vi "CraciunAlexandru_ChelaruIoana_FSM_3a (1).vi"() -> ()   [LabVIEW 2021]
uses:
  <vilib>/Skyline/Tag/Shared/typedefs/DataType.ctl
  <vilib>/Skyline/Configuration/Configuration HTTP_class/Open Configuration HTTP Auto.vi
  <vilib>/Skyline/Tag/Wrapper/Wrapper_class/Write Tag (I32).vi
  <vilib>/Skyline/Tag/Wrapper/Wrapper HTTP_class/NI Skyline Tag HTTP.lvclass
  <vilib>/Skyline/Tag/Shared/NI Skyline Tag.lvlib
  <vilib>/Skyline/Configuration/Configuration HTTP_class/NI Skyline Configuration HTTP.lvclass
  <vilib>/Skyline/Tag/Wrapper/Wrapper_class/NI Skyline Tag.lvclass
panel:
  in  "?":bool
  out "Time loading":u8(slide) scale=0.0..100.0
  in  "?":bool
  out "Electronics received":bool
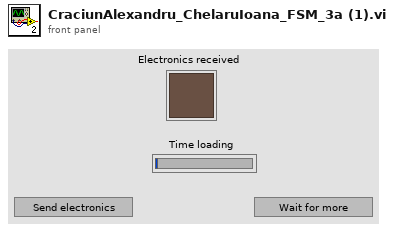
[diagram p1: front panel]
types:
  T1 = enum16{"PromtQuestion", "Wait", "RequestAnswear", "Done"}
  T2 = typedef "NI Skyline Tag.lvlib/DataType.ctl" = enum32{"Double", "I32", "String", "Boolean", "U64", "Timestamp"}
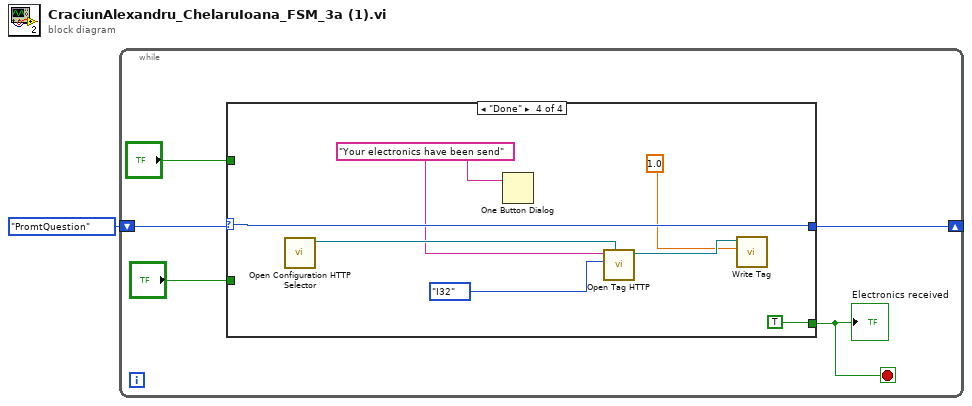
[diagram p0: block diagram]
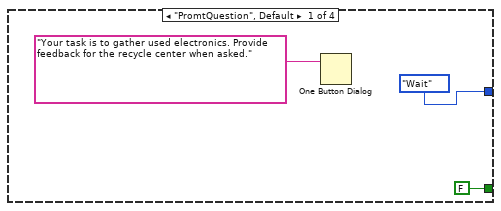
[diagram p2: hidden frame]
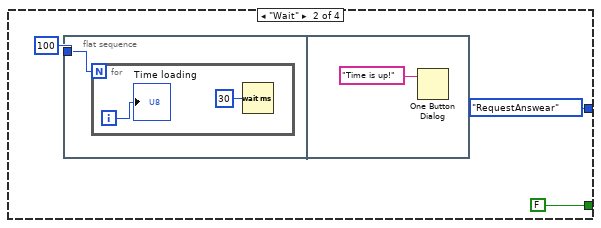
[diagram p3: hidden frame]
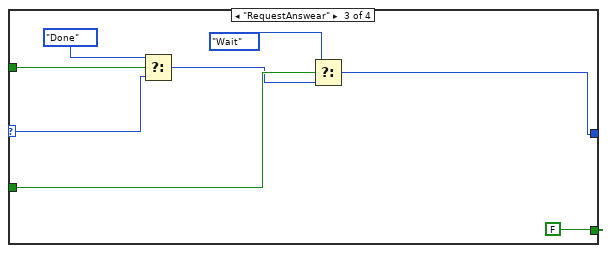
[diagram p4: hidden frame]
diagram:
  n1 = while {
    shift-right: [w4] -> _
    shift-left: T1."PromtQuestion" -> [w6]
    stop <- w5 stop-if-true
    n2 = case shown="\"Done\"" w6 {
      selector: w6 -> [_ _ w22 w31]
      tunnel: [FALSE FALSE FALSE TRUE] -> w5
      tunnel: [T1."Wait" T1."RequestAnswear" w19 w31] -> w4
      tunnel: "?" -> [_ _ w24 _]
      tunnel: "?" -> [_ _ w21 _]
      frame "PromtQuestion", Default {
        n3 = One Button Dialog(message="Your task is to gather used electronics. Provide feedback for the recycle center when asked.") -> ()  [unwired: 1 in, 1 out]
      }
      frame "Wait" {
        n4 = flat-sequence {
          tunnel: 100 -> [w13]
          frame #0 {
            n5 = for {
              N: w13 -> [_]
              i -> [w14]
              n6 = Wait (ms)(milliseconds to wait=u32 30) -> ()  [unwired: 1 out]
              "Time loading" <- w14
            }
          }
          frame #1 {
            n7 = One Button Dialog(message="Time is up!" ("Teacher is thinking!")) -> ()  [unwired: 1 in, 1 out]
          }
        }
      }
      frame "RequestAnswear" {
        n8 = Select(t=T1."Done", s=w24, f=w22) -> (s? t:f=w20:T1)
        n9 = Select(t=T1."Wait", s=w21, f=w20) -> (s? t:f=w19:T1)
      }
      frame "Done" {
        w27 = "Your electronics have been send" ("message")
        n10 = call-poly <vilib>:"Open Configuration HTTP Selector.vi"() -> ("configuration"=w28:refnum<class "NI Skyline Configuration HTTP.lvclass">)  [unwired: 10 in, 1 out]
        n11 = One Button Dialog(message=w27) -> ()  [unwired: 1 in, 1 out]
        n12 = call <vilib>:"Open Tag HTTP.vi"("configuration"=w28, "Data Type"=DataType."I32", "path"=w27) -> ("tag"=w26:refnum<class "NI Skyline Tag.lvclass">)  [unwired: 7 in, 1 out]
        n13 = call-poly <vilib>:"Write Tag.vi"("value"=1.0, "tag in"=w26) -> ()  [unwired: 8 in, 2 out]
      }
    }
    "Electronics received" <- w5
  }
